vi "Waveform - Create.vi"() -> ()   [LabVIEW 2020]
doc: "Shows how to create a waveform with an array of random numbers as input."
panel:
  out "Waveform":waveform(dbl)
  out "Waveform Graph":waveform(dbl)(graph)
  # "Overview: Demonstrates how to create a waveform data type with the Build Waveform and Set Waveform Attribute functions.\nInstructions:\nRun the VI. A waveform data type is created from scratch. See the block diagram for more information."
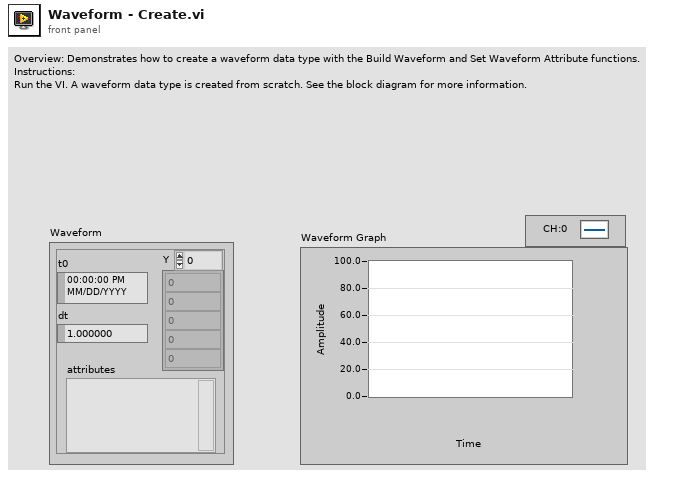
[diagram p1: front panel]
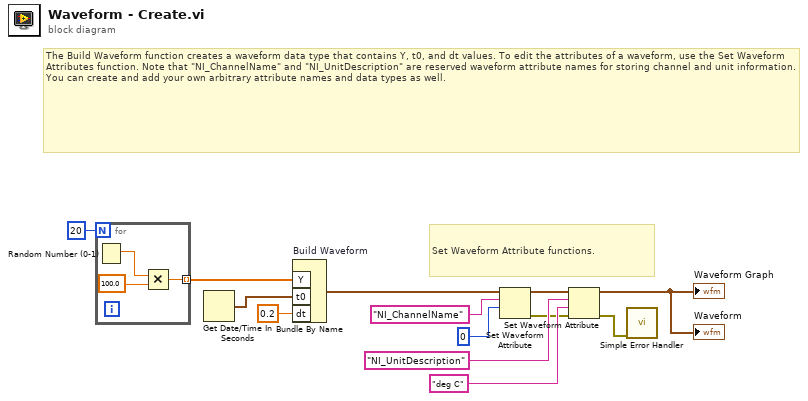
[diagram p0: block diagram]
diagram:
  # "The Build Waveform function creates a waveform data type that contains Y, t0, and dt values. To edit the attributes of a waveform, use the Set Waveform Attributes function. Note that \"NI_ChannelName\" and \"NI_UnitDescription\" are reserved waveform attribute names for storing channel and unit information. You can create and add your own arbitrary attribute names and data types as well."
  # "Set Waveform Attribute functions."
  n1 = for {
    N: 20 ("# points") -> [_]
    tunnel: [w15] -> w7 mode=indexing
    n2 = Random Number (0-1)() -> (number: 0 to 1=w16:dbl)
    n3 = Multiply(x=w16, y=100.0) -> (x*y=w15:dbl)
  }
  n4 = Get Date/Time In Seconds() -> (seconds since 1Jan1904=w5:timestamp)
  n5 = Bundle By Name "Build Waveform"("Y"=w7, "t0"=w5, "dt"=0.2) -> (w12:waveform(dbl))  [unwired: 1 in]
  n6 = Set Waveform Attribute(5:0 ("channel #"), 6:"NI_ChannelName" ("Channel Name"), 7:w12) -> (0:w3:errorcluster, 3:w9:waveform(dbl))  [unwired: 1 in, 1 out]
  n7 = Set Waveform Attribute(4:w3, 5:"deg C" ("channel unit"), 6:"NI_UnitDescription" ("Channel Unit"), 7:w9) -> (0:w2:errorcluster, 3:→"Waveform Graph" →"Waveform":waveform(dbl))  [unwired: 1 out]
  n8 = call <vilib>:"Simple Error Handler.vi"("error in (no error)"=w2) -> ()  [unwired: 4 in, 5 out]
